vi "Register.vi"(7 "Event":refnum<class "Event.lvclass">, 8 "Error In":errorcluster, 9 "Event Handler Msg":refnum<class "Event Generated Msg.lvclass">, 10 "Registrant Enq":refnum<class "Message Enqueuer.lvclass">, 11 "Event Source In":refnum<class "Event Source.lvclass">) -> (0 "Error Out":errorcluster, 3 "Event Source Out":refnum<class "Event Source.lvclass">)   [LabVIEW 2019, in "Event Source.lvlib" / "Event Source.lvclass"]
doc: "This method registers a specific Actors Enqueuer and a Zero Coupling based message (inheriting from Event Generated Msg.lvclass) to used when the specified Event is Fired anywhere inside the Event Source Actor."
uses:
  Event Source.lvclass
  Event/Event.lvclass
  Event/Event.lvclass/Event.ctl
  Event Source.lvclass/Event Source.ctl
  <resource>/AFDebug/AF Debug.lvlib
  <vilib>/Utility/miscctls.llb/LVMapReplaceAction.ctl
  Event Source Messages/Event Generated Msg/Event Generated Msg.lvclass
  <vilib>/ActorFramework/Message Enqueuer/Message Enqueuer.lvclass
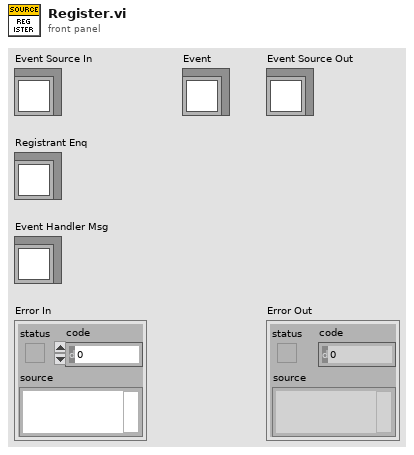
[diagram p1: front panel]
types:
  T1 = typedef "LVMapReplaceAction.ctl" = enum32{"Modify Entry only if found", "Add or Modify Entry", "Delete Entry"}
  T2 = map{string, map{refnum<class "Message Enqueuer.lvclass">, refnum<class "Event Generated Msg.lvclass">}}
  T3 = map{refnum<class "Message Enqueuer.lvclass">, refnum<class "Event Generated Msg.lvclass">}
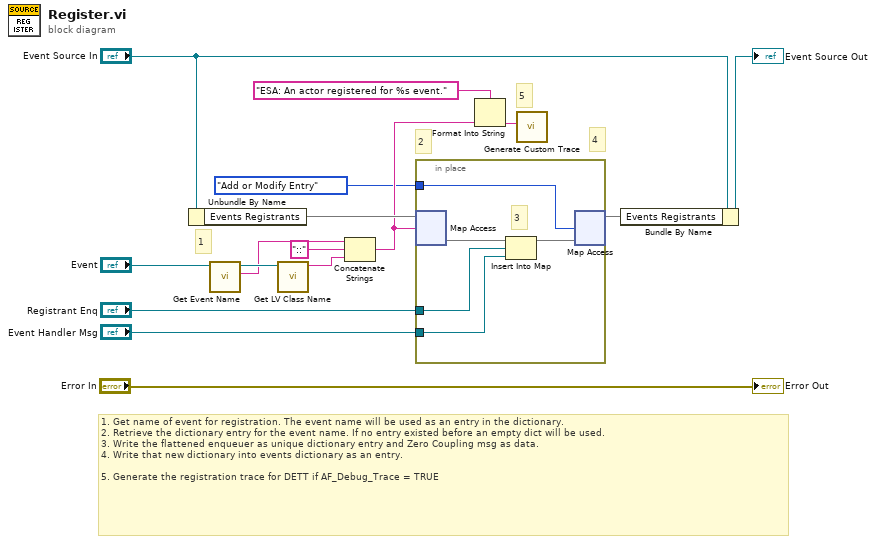
[diagram p0: block diagram]
diagram:
  # "5"
  # "4"
  # "2"
  # "1"
  # "1. Get name of event for registration. The event name will be used as an entry in the dictionary.\n2. Retrieve the dictionary entry for the event name. If no entry existed before an empty dict will be used.\n3. Write the flattened enqueuer as unique dictionary entry and Zero Coupling msg as data.\n4. Write that new dictionary into events dictionary as an entry.\n\n5. Generate the registration trace for DETT if AF_Debug_Trace = TRUE"
  n1 = Unbundle By Name("Event Source In") -> ("Events Registrants"=w5:T2)
  n2 = call "Get Event Name.vi"("Event In"="Event") -> ("Name"=w6:string, "Event Out"=w9:refnum<class "Event.lvclass">)  [unwired: 9 in]
  n3 = call <vilib>:"Get LV Class Name.vi"("object"=w9) -> ("class name"=w7:string)  [unwired: 9 in, 1 out]
  n4 = Concatenate Strings(w6, "::" ("string"), w7) -> (w4:string)
  n5 = in-place {
    in-place-border: "Registrant Enq" -> [w19]
    in-place-border: "Event Handler Msg" -> [w18]
    in-place-border: LVMapReplaceAction."Add or Modify Entry" ("action") -> [w17]
    # "3"
    n6 = in-place-map #1(w5, w4) -> (w21:T3)  [unwired: 1 in, 1 out]
    n7 = Insert Into Map(map in=w21, key=w19, value=w18) -> (map out=w20:T3)  [unwired: 2 out]
    n8 = in-place-map #1(w20, w17) -> (w2:T2)  [unwired: 2 out]
  }
  n9 = Format Into String(format string="ESA: An actor registered for %s event." ("Custom Action"), w4) -> (resulting string=w10:string)  [unwired: 2 in, 1 out]
  n10 = call <resource>:"Generate Custom Trace.vi"("Custom Action"=w10) -> ()  [unwired: 11 in]
  n11 = Bundle By Name(cluster="Event Source In", "Events Registrants"=w2) -> (→"Event Source Out":refnum<class "Event Source.lvclass">)
  "Error Out" <- "Error In"
